vi "initIP.vi"() -> ()   [LabVIEW 2010]
uses:
  GlobalCostants.vi
panel:
  in  "PortIPList":string[](array[string])=["040000000000", "030000000000", "010000000000", "020000000000"]
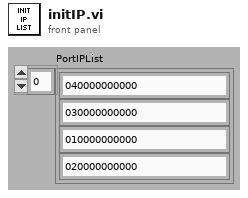
[diagram p1: front panel]
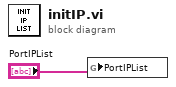
[diagram p0: block diagram]
diagram:
  n1 = global write "GlobalCostants.vi" "PortIPList"("PortIPList") -> ()
